vi "CMD_Harvest.vi"(1 "Line":string) -> (0 "Done":bool)   [LabVIEW 2017, in "Apple script.lvlib"]
uses:
  Apple script.lvlib
panel:
  in  "Parameters":i32[](array[numeric])=[1]
  in  "Subcommands":string[](array[string])=["for", "in", "out"]
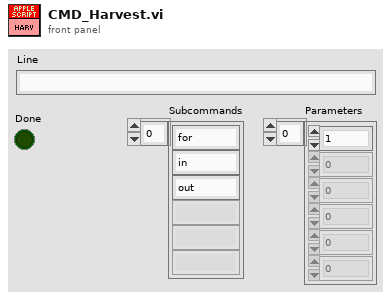
[diagram p1: front panel]
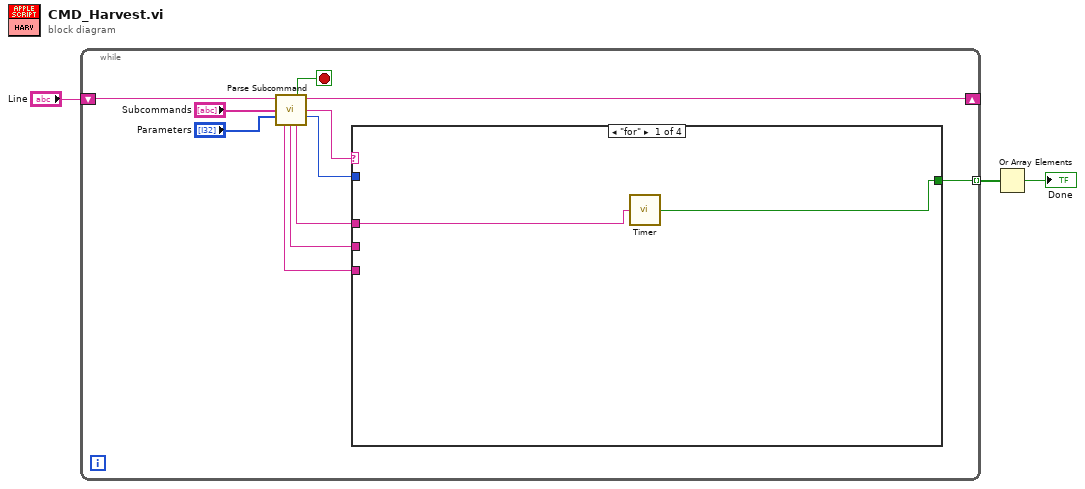
[diagram p0: block diagram]
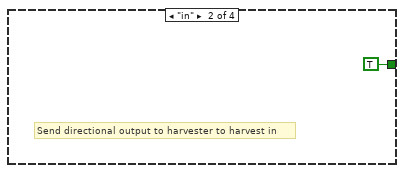
[diagram p2: hidden frame]
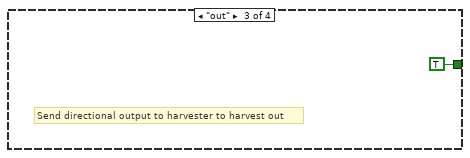
[diagram p3: hidden frame]
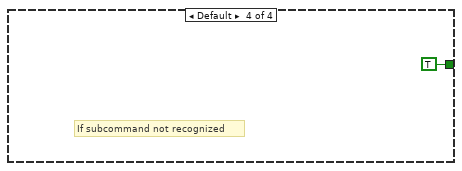
[diagram p4: hidden frame]
diagram:
  n1 = while {
    shift-right: [w11] -> _
    shift-left: "Line" -> [w14]
    tunnel: [w4] -> w2 mode=indexing
    stop <- w10 stop-if-true
    n2 = call "Parse Subcommand.vi"("Text In"=w14, "Subcommands"="Subcommands", "Parameters"="Parameters") -> ("Done"=w10:bool, "Text Out"=w11:string, "Subcommand"=w9:string, "# of Parameters"=w8:i32, "Parameter 3"=w5:string, "Parameter 2"=w6:string, "Parameter 1"=w7:string)  [unwired: 6 in]
    n3 = case shown="\"for\"" w9 {
      tunnel: w8 -> [_ _ _ _]
      tunnel: w7 -> [w16 _ _ _]
      tunnel: w6 -> [_ _ _ _]
      tunnel: w5 -> [_ _ _ _]
      tunnel: [w15 TRUE ("Done") TRUE ("Done") TRUE] -> w4
      frame "for" {
        n4 = call "Timer.vi"("Seconds (string)"=w16) -> ("Done"=w15:bool)
      }
      frame "in" {
        # "Send directional output to harvester to harvest in"
      }
      frame "out" {
        # "Send directional output to harvester to harvest out"
      }
      frame Default {
        # "If subcommand not recognized"
      }
    }
  }
  n5 = Or Array Elements(Boolean array=w2) -> (logical OR=→"Done":bool)
